vi "Enqueue Return Value.vi"(8 "error in (no error)":errorcluster, 10 "Indicator Values":cluster{"Name":string, "Variant Data":variant}[](array[cluster]), 11 "Mock In":refnum<class "LMock Mock.lvclass">) -> (0 "error out":errorcluster, 3 "Mock Out":refnum<class "LMock Mock.lvclass">)   [LabVIEW 2020, in "LMock Mock.lvclass"]
uses:
  LMock Mock.lvclass
  LMock Mock.lvclass/LMock Mock.ctl
  Core/VI Call/VI Call.lvclass
  Parametric VI Call/Parametric VI Call.lvclass
  C:/git/astemes-lmock/source/Core/VI Call/VI Call.lvclass
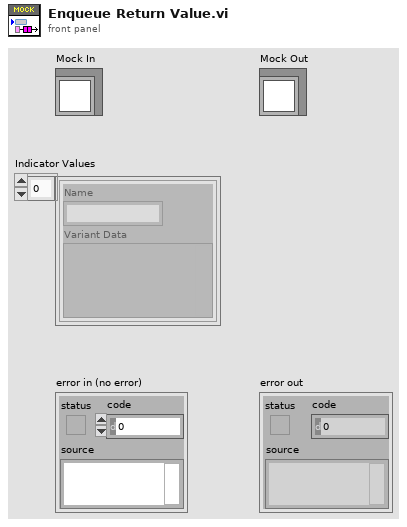
[diagram p1: front panel]
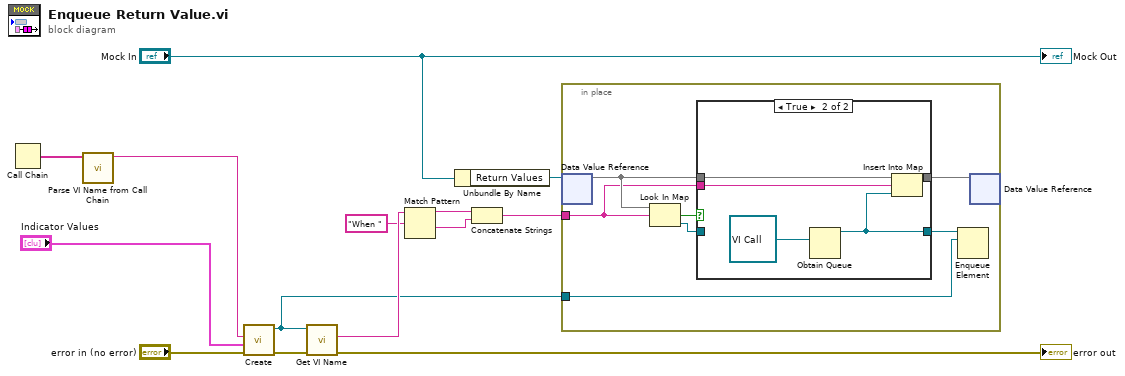
[diagram p0: block diagram]
diagram:
  n1 = Call Chain() -> (call chain=w2:string[])
  n2 = call "Parse VI Name from Call Chain.vi"("call chain"=w2) -> ("VI Name"=w1:string)  [unwired: 10 in]
  n3 = call "Create.vi"("error in (no error)"="error in (no error)", "Control Values"="Indicator Values", "VI Name"=w1) -> ("error out"=w13:errorcluster, "Parametric VI Call Out"=w4:refnum<class "Parametric VI Call.lvclass">)  [unwired: 7 in]
  n4 = call-dynamic "Get VI Name.vi"("error in (no error)"=w13, "Parametric VI Call In"=w4) -> ("error out"=→"error out":errorcluster, "VI Name"=w11:string)  [unwired: 8 in]
  n5 = Match Pattern(string=w11, regular expression="When ") -> (before substring=w9:string, after substring=w8:string)  [unwired: 1 in, 2 out]
  n6 = Unbundle By Name("Mock In") -> ("Return Values"=w6:refnum<data-value>)
  n7 = Concatenate Strings(w9, w8) -> (w5:string)
  n8 = in-place {
    in-place-border: w5 -> [w18]
    in-place-border: w4 -> [w15]
    n9 = in-place-dvr #1(w6) -> (w20:map{string, refnum<queue>})  [unwired: 1 out]
    n10 = Look In Map(map=w20, key=w18) -> (key not found?=w21:bool, value=w19:refnum<queue>)  [unwired: 1 in]
    n11 = case shown="True" w21 {
      tunnel: w20 -> [w23 w27]
      tunnel: w19 -> [w22 _]
      tunnel: w18 -> [_ w26]
      tunnel: [w23 w25] -> w17
      tunnel: [w22 w24] -> w16
      frame False {
      }
      frame True {
        n12 = Obtain Queue(element data type=refnum<class "VI Call.lvclass"> refnum ("Call Out")) -> (queue out=w24:refnum<queue>)  [unwired: 4 in, 2 out]
        n13 = Insert Into Map(map in=w27, key=w26, value=w24) -> (map out=w25:map{string, refnum<queue>})  [unwired: 2 out]
      }
    }
    n14 = Enqueue Element(queue=w16, element=w15) -> ()  [unwired: 2 in, 3 out]
    n15 = in-place-dvr #1(w17) -> ()  [unwired: 2 out]
  }
  "Mock Out" <- "Mock In"
